vi "WSVCAP SHL FPGA LL Enumeration Builder.vi"() -> ()   [LabVIEW 2017]
uses:
  Type Defs/WSVCAP SHL Procedure Enum.ctl
  Type Defs/WSVCAP SHL Transaction I2C-Write Enum.ctl
  Type Defs/WSVCAP SHL Operation I2C-Send Slave Address Enum.ctl
  Type Defs/WSVCAP SHL Operation I2C-Send Sub Address Enum.ctl
  Type Defs/WSVCAP SHL Operation I2C-Send Data Bytes Enum.ctl
  Type Defs/WSVCAP SHL I2C Read Data Bytes Enum.ctl
  Type Defs/WSVCAP SHL I2C Read Data Transaction Enum.ctl
  Type Defs/WSVCAP SHL Procedure I2C-Send Start or Stop Sequence Enum.ctl
  Type Defs/WSVCAP SHL Procedure I2C-Send Address Byte Enum.ctl
  Type Defs/WSVCAP SHL Procedure I2C-Receive Byte Enum.ctl
  Type Defs/WSVCAP SHL I2C Read ACK Enum.ctl
  Type Defs/WSVCAP SHL Procedure I2C-Write ACK Enum.ctl
  Type Defs/WSVCAP SHL Procedure I2C-Send Data Byte Enum.ctl
  Type Defs/WSVCAP SHL Operation SPI-Send Receive Enum.ctl
  Type Defs/WSVCAP SHL Procedure SPI-Send Receive  Data Enum.ctl
  Type Defs/WSVCAP SHL Transaction SPI Write_Read Enum.ctl
panel:
  in  "Procedure":T1
  in  "Procedure Step":T2(ring)
  in  "Operation Step":T3(ring)
  in  "Transaction Step":T4(ring)
  in  "TR:SPI-Write/Read Data":T5
  in  "PRC:SPI-Send/Receive Data":T6=enum."2: Wait"
  in  "OP:SPI-Write/Read Data":T7
  in  "PRC:Send Data Byte":T8=enum."9: Check Bits Remaining"
  in  "PRC:Write ACK":T9=enum."3: Set Clock High"
  in  "PRC:Read ACK":T10=enum."3: Read ACK Bit"
  in  "PRC:Receive Byte":T11=enum."8: Wait"
  in  "PRC:Send Address Byte":T12=enum."8: Check Bits Remaining"
  in  "PRC:Send Start/Stop Sequence":T13
  in  "TR:I2C-Read Data":T14=enum."IV:Read Data Bytes"
  in  "OP:Read Data Bytes":T15
  in  "OP:Send Data Bytes":T16
  in  "OP:Send Sub Address":T17
  in  "OP:Send Slave Address":T18
  in  "TR:I2C-Write Data":T19
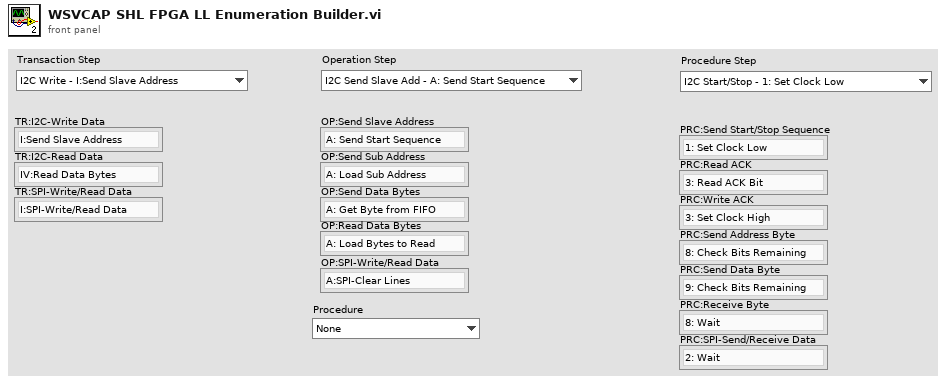
[diagram p1: front panel]
types:
  T1 = typedef "WSVCAP SHL Procedure Enum.ctl" = enum16{"None", "I2C-Send Start/Stop Sequence", "I2C-Send Address Byte", "I2C-Send Data Byte", "I2C-Read ACK", "I2C-Receive Byte", "I2C-Write ACK", "RFFE-Clear Lines", "RFFE-Send SSC", "RFFE-Send Data", "RFFE-Receive Data", "RFFE-Wait CMD Delay", "SRL-Clear Lines", "SRL-Send Data", "SRL-Wait CMD Delay"}
  T2 = enum16{"I2C Start/Stop - 1: Set Clock Low", "I2C Start/Stop - 2: Wait", "I2C Start/Stop - 3: Set Data I", "I2C Start/Stop - 4: Wait", "I2C Start/Stop - 5: Set Clock High", "I2C Start/Stop - 6: Wait", "I2C Start/Stop - 7: Set Data II", "I2C Start/Stop - 8: Wait", "I2C Start/Stop - 9: Set Clock Low", "I2C Start/Stop - 10: Wait", "I2C Read ACK - 1: Set Clock High", "I2C Read ACK - 2: Wait", "I2C Read ACK - 3: Read ACK Bit", "I2C Read ACK - 4: Wait", "I2C Read ACK - 5: Set Clock Low", "I2C Read ACK - 6: Wait", "I2C Write ACK - 1: Write ACK Bit", "I2C Write ACK - 2: Wait", "I2C Write ACK - 3: Set Clock High", "I2C Write ACK - 4: Wait", "I2C Write ACK - 5: Set Clock Low", "I2C Write ACK - 6: Wait", "I2C Write ACK - 7: Set Data Low", "I2C Send Add - 1: Reset Bits Remaining", "I2C Send Add - 2: Set Data Bit", "I2C Send Add - 3: Wait", "I2C Send Add - 4: Set Clock High", "I2C Send Add - 5: Wait", "I2C Send Add - 6: Set Clock Low", "I2C Send Add - 7: Wait", "I2C Send Add - 8: Check Bits Remaining", "I2C Send Data - 1: Reset Bits Remaining", "I2C Send Data - 2: Load Write Bit from FIFO", "I2C Send Data - 3: Set Data Bit", "I2C Send Data - 4: Wait", "I2C Send Data - 5: Set Clock High", "I2C Send Data - 6: Wait", "I2C Send Data - 7: Set Clock Low", "I2C Send Data - 8: Wait", "I2C Send Data - 9: Check Bits Remaining", "I2C Receive Data - 1: Reset Bits Remaining", "I2C Receive Data - 2: Wait", "I2C Receive Data - 3: Set Clock High", "I2C Receive Data - 4: Wait", "I2C Receive Data - 5: Read Data Bit", "I2C Receive Data - 6: Wait", "I2C Receive Data - 7: Set Clock Low", "I2C Receive Data - 8: Wait", "I2C Receive Data - 9: Check Bits Remaining", "SPI Send/Receive - 1: Load SDA - Clock Low", "SPI Send/Receive - 2: Wait", "SPI Send/Receive - 3: Load DATO - Clock High", "SPI Send/Receive - 4: Wait"}
  T3 = enum16{"I2C Send Slave Add - A: Send Start Sequence", "I2C Send Slave Add - B: Load Address Byte", "I2C Send Slave Add - C: Send Address Byte", "I2C Send Slave Add - D: Read Slave ACK", "I2C Send Sub Add - A: Load Sub Address", "I2C Send Sub Add - B: Send Address Byte", "I2C Send Sub Add - C: Read Slave ACK", "I2C Send Data - A: Get Byte from FIFO", "I2C Send Data - B: Send Data Byte", "I2C Send Data - C: Read Slave ACK", "I2C Send Data - D: Send Stop Sequence", "I2C Read Data - A: Load Bytes to Read", "I2C Read Data - B: Receive Byte", "I2C Read Data - C: Write Master ACK", "I2C Read Data - D: Send Stop Sequence", "SPI Write/Read - A:SPI-Clear Lines", "SPI Write/Read - B:SPI-Send/Receive Data", "SPI Write/Read - C: SPI-Wait CMD Delay", "SPI Write/Read - D:SPI-Clear Lines"}
  T4 = enum16{"I2C Write - I:Send Slave Address", "I2C Write - II:Send Sub Address", "I2C Write - III:Send Data Bytes", "I2C Read - I:Send Slave Address (W)", "I2C Read - II:Send Sub Address", "I2C Read - III:Send Slave Address (R)", "I2C Read - IV:Read Data Bytes", "SPI Write/Read - I:SPI-Write/Read Data"}
  T5 = typedef "WSVCAP SHL Transaction SPI Write_Read Enum.ctl" = enum16{"I:SPI-Write/Read Data"}
  T6 = typedef "WSVCAP SHL Procedure SPI-Send Receive  Data Enum.ctl" = enum16{"1: Load SDA - Clock Low", "2: Wait", "3: Load DATO - Clock High", "4: Wait"}
  T7 = typedef "WSVCAP SHL Operation SPI-Send Receive Enum.ctl" = enum16{"A:SPI-Clear Lines", "B:SPI-Send/Receive Data", "C: SPI-Wait CMD Delay", "D:SPI-Clear Lines"}
  T8 = typedef "WSVCAP SHL Procedure I2C-Send Data Byte Enum.ctl" = enum16{"1: Reset Bits Remaining", "2: Load Write Bit from FIFO", "3: Set Data Bit", "4: Wait", "5: Set Clock High", "6: Wait", "7: Set Clock Low", "8: Wait", "9: Check Bits Remaining"}
  T9 = typedef "WSVCAP SHL Procedure I2C-Write ACK Enum.ctl" = enum16{"1: Write ACK Bit", "2: Wait", "3: Set Clock High", "4: Wait", "5: Set Clock Low", "6: Wait", "7: Set Data Low"}
  T10 = typedef "WSVCAP SHL I2C Read ACK Enum.ctl" = enum16{"1: Set Clock High", "2: Wait", "3: Read ACK Bit", "4: Wait", "5: Set Clock Low", "6: Wait"}
  T11 = typedef "WSVCAP SHL Procedure I2C-Receive Byte Enum.ctl" = enum16{"1: Reset Bits Remaining", "2: Wait", "3: Set Clock High", "4: Wait", "5: Read Data Bit", "6: Wait", "7: Set Clock Low", "8: Wait", "9: Check Bits Remaining"}
  T12 = typedef "WSVCAP SHL Procedure I2C-Send Address Byte Enum.ctl" = enum16{"1: Reset Bits Remaining", "2: Set Data Bit", "3: Wait", "4: Set Clock High", "5: Wait", "6: Set Clock Low", "7: Wait", "8: Check Bits Remaining"}
  T13 = typedef "WSVCAP SHL Procedure I2C-Send Start or Stop Sequence Enum.ctl" = enum16{"1: Set Clock Low", "2: Wait", "3: Set Data I", "4: Wait", "5: Set Clock High", "6: Wait", "7: Set Data II", "8: Wait", "9: Set Clock Low", "10: Wait"}
  T14 = typedef "WSVCAP SHL I2C Read Data Transaction Enum.ctl" = enum16{"I:Send Slave Address (W)", "II:Send Sub Address", "III:Send Slave Address (R)", "IV:Read Data Bytes"}
  T15 = typedef "WSVCAP SHL I2C Read Data Bytes Enum.ctl" = enum16{"A: Load Bytes to Read", "B: Receive Byte", "C: Write Master ACK", "D: Send Stop Sequence"}
  T16 = typedef "WSVCAP SHL Operation I2C-Send Data Bytes Enum.ctl" = enum16{"A: Get Byte from FIFO", "B: Send Data Byte", "C: Read Slave ACK", "D: Send Stop Sequence"}
  T17 = typedef "WSVCAP SHL Operation I2C-Send Sub Address Enum.ctl" = enum16{"A: Load Sub Address", "B: Send Address Byte", "C: Read Slave ACK"}
  T18 = typedef "WSVCAP SHL Operation I2C-Send Slave Address Enum.ctl" = enum16{"A: Send Start Sequence", "B: Load Address Byte", "C: Send Address Byte", "D: Read Slave ACK"}
  T19 = typedef "WSVCAP SHL Transaction I2C-Write Enum.ctl" = enum16{"I:Send Slave Address", "II:Send Sub Address", "III:Send Data Bytes"}
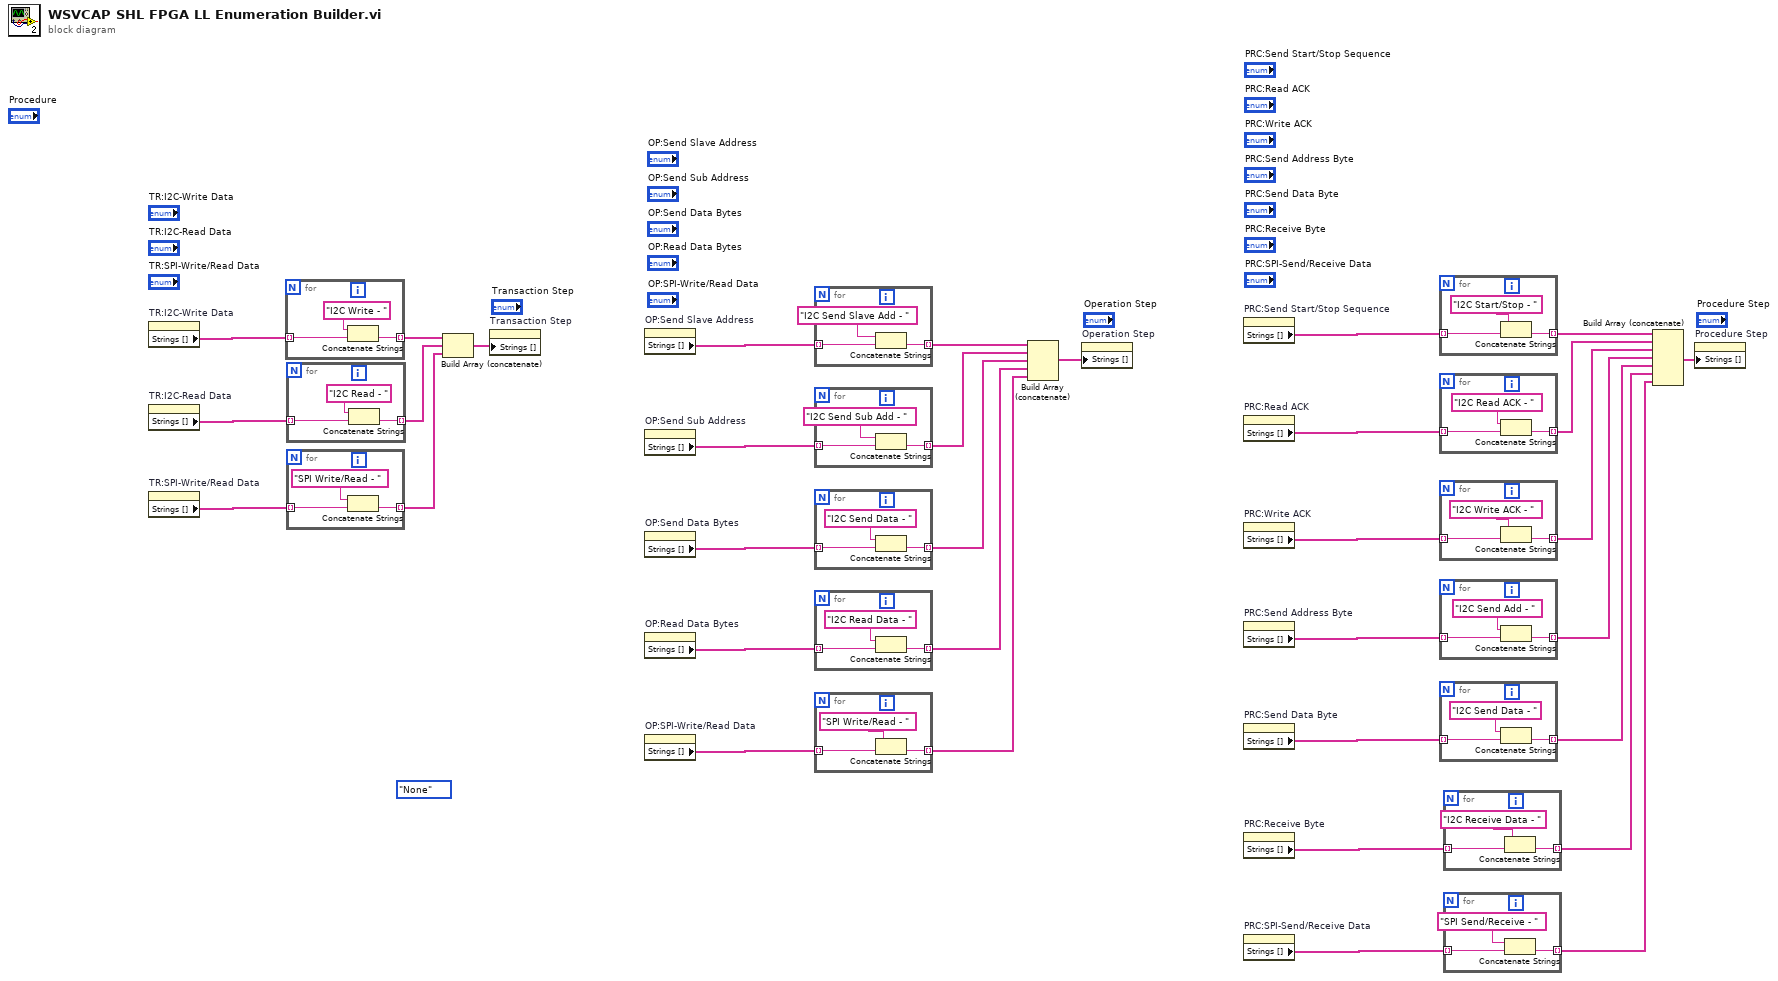
[diagram p0: block diagram]
diagram:
  (unwired) WSVCAP_SHL_Procedure_Enum."None" ("Procedure")
  n1 = property on="TR:I2C-Write Data" class="Enum (strict)"() -> ("Strings []"=w33:string[])  [unwired: 2 in, 2 out]
  n2 = property on="TR:I2C-Read Data" class="Enum (strict)"() -> ("Strings []"=w31:string[])  [unwired: 2 in, 2 out]
  n3 = property on="TR:SPI-Write/Read Data" class="Enum (strict)"() -> ("Strings []"=w29:string[])  [unwired: 2 in, 2 out]
  n4 = for {
    tunnel: [w34] -> w32 mode=indexing
    tunnel: w33 -> [w36] mode=indexing
    n5 = Concatenate Strings("I2C Write - " ("string"), w36) -> (w34:string)
  }
  n6 = for {
    tunnel: [w37] -> w30 mode=indexing
    tunnel: w31 -> [w39] mode=indexing
    n7 = Concatenate Strings("I2C Read - " ("string"), w39) -> (w37:string)
  }
  n8 = for {
    tunnel: [w40] -> w28 mode=indexing
    tunnel: w29 -> [w42] mode=indexing
    n9 = Concatenate Strings("SPI Write/Read - " ("string"), w42) -> (w40:string)
  }
  n10 = Build Array (concatenate)(w32, w30, w28) -> (w27:string[])
  n11 = property on="Transaction Step" class="Enum (strict)"("Strings []"=w27) -> ()  [unwired: 2 in, 2 out]
  n12 = property on="OP:Send Slave Address" class="Enum (strict)"() -> ("Strings []"=w26:string[])  [unwired: 2 in, 2 out]
  n13 = property on="OP:Send Sub Address" class="Enum (strict)"() -> ("Strings []"=w25:string[])  [unwired: 2 in, 2 out]
  n14 = property on="OP:Send Data Bytes" class="Enum (strict)"() -> ("Strings []"=w24:string[])  [unwired: 2 in, 2 out]
  n15 = property on="OP:Read Data Bytes" class="Enum (strict)"() -> ("Strings []"=w23:string[])  [unwired: 2 in, 2 out]
  n16 = property on="OP:SPI-Write/Read Data" class="Enum (strict)"() -> ("Strings []"=w22:string[])  [unwired: 2 in, 2 out]
  n17 = for {
    tunnel: [w43] -> w21 mode=indexing
    tunnel: w26 -> [w45] mode=indexing
    n18 = Concatenate Strings("I2C Send Slave Add - " ("string"), w45) -> (w43:string)
  }
  n19 = for {
    tunnel: [w46] -> w20 mode=indexing
    tunnel: w25 -> [w48] mode=indexing
    n20 = Concatenate Strings("I2C Send Sub Add - " ("string"), w48) -> (w46:string)
  }
  n21 = for {
    tunnel: [w49] -> w19 mode=indexing
    tunnel: w24 -> [w51] mode=indexing
    n22 = Concatenate Strings("I2C Send Data - " ("string"), w51) -> (w49:string)
  }
  n23 = for {
    tunnel: [w52] -> w18 mode=indexing
    tunnel: w23 -> [w54] mode=indexing
    n24 = Concatenate Strings("I2C Read Data - " ("string"), w54) -> (w52:string)
  }
  n25 = for {
    tunnel: [w55] -> w17 mode=indexing
    tunnel: w22 -> [w57] mode=indexing
    n26 = Concatenate Strings("SPI Write/Read - " ("string"), w57) -> (w55:string)
  }
  n27 = Build Array (concatenate)(w21, w20, w19, w18, w17) -> (w2:string[])
  n28 = property on="Operation Step" class="Enum (strict)"("Strings []"=w2) -> ()  [unwired: 2 in, 2 out]
  n29 = property on="PRC:Send Start/Stop Sequence" class="Enum (strict)"() -> ("Strings []"=w9:string[])  [unwired: 2 in, 2 out]
  n30 = property on="PRC:Read ACK" class="Enum (strict)"() -> ("Strings []"=w8:string[])  [unwired: 2 in, 2 out]
  n31 = property on="PRC:Write ACK" class="Enum (strict)"() -> ("Strings []"=w7:string[])  [unwired: 2 in, 2 out]
  n32 = property on="PRC:Send Address Byte" class="Enum (strict)"() -> ("Strings []"=w6:string[])  [unwired: 2 in, 2 out]
  n33 = property on="PRC:Send Data Byte" class="Enum (strict)"() -> ("Strings []"=w5:string[])  [unwired: 2 in, 2 out]
  n34 = property on="PRC:Receive Byte" class="Enum (strict)"() -> ("Strings []"=w4:string[])  [unwired: 2 in, 2 out]
  n35 = property on="PRC:SPI-Send/Receive Data" class="Enum (strict)"() -> ("Strings []"=w3:string[])  [unwired: 2 in, 2 out]
  n36 = for {
    tunnel: [w58] -> w12 mode=indexing
    tunnel: w9 -> [w60] mode=indexing
    n37 = Concatenate Strings("I2C Start/Stop - " ("string"), w60) -> (w58:string)
  }
  n38 = for {
    tunnel: [w61] -> w13 mode=indexing
    tunnel: w8 -> [w63] mode=indexing
    n39 = Concatenate Strings("I2C Read ACK - " ("string"), w63) -> (w61:string)
  }
  n40 = for {
    tunnel: [w64] -> w14 mode=indexing
    tunnel: w7 -> [w66] mode=indexing
    n41 = Concatenate Strings("I2C Write ACK - " ("string"), w66) -> (w64:string)
  }
  n42 = for {
    tunnel: [w67] -> w15 mode=indexing
    tunnel: w6 -> [w69] mode=indexing
    n43 = Concatenate Strings("I2C Send Add - " ("string"), w69) -> (w67:string)
  }
  n44 = for {
    tunnel: [w70] -> w16 mode=indexing
    tunnel: w5 -> [w72] mode=indexing
    n45 = Concatenate Strings("I2C Send Data - " ("string"), w72) -> (w70:string)
  }
  n46 = for {
    tunnel: [w73] -> w11 mode=indexing
    tunnel: w4 -> [w75] mode=indexing
    n47 = Concatenate Strings("I2C Receive Data - " ("string"), w75) -> (w73:string)
  }
  n48 = for {
    tunnel: [w76] -> w10 mode=indexing
    tunnel: w3 -> [w78] mode=indexing
    n49 = Concatenate Strings("SPI Send/Receive - " ("string"), w78) -> (w76:string)
  }
  n50 = Build Array (concatenate)(w12, w13, w14, w15, w16, w11, w10) -> (w1:string[])
  n51 = property on="Procedure Step" class="Enum (strict)"("Strings []"=w1) -> ()  [unwired: 2 in, 2 out]
